vi "AddClassCase.vi"(2 "error in":errorcluster, 3 "Class path":path, 4 "CaseSel Refnum":refnum<vi>) -> (0 "error out":errorcluster, 1 "dup CaseSel Refnum":refnum<vi>)   [LabVIEW 2009, in "HGF_VisitorGenerator.lvlib"]
doc: "add case with default object of given class to factory's classes.vi"
uses:
  HGF_VisitorGenerator.lvlib
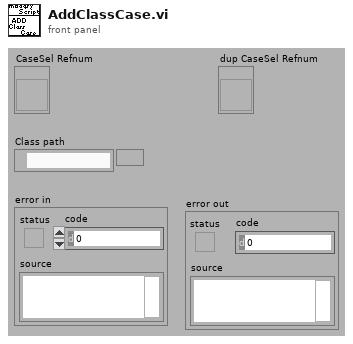
[diagram p1: front panel]
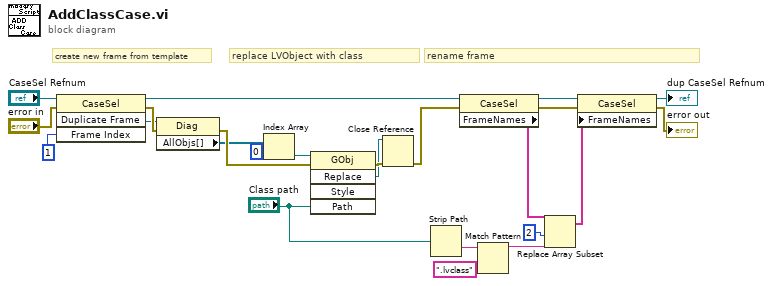
[diagram p0: block diagram]
diagram:
  # "rename frame"
  # "replace LVObject with class"
  # "create new frame from template"
  n1 = invoke class="CaseSel" method="Duplicate Frame"(reference="CaseSel Refnum", error in="error in", "Frame Index"=u32 1) -> (reference out=w8:refnum<vi>, error out=w23:errorcluster, "Duplicate Frame"=w21:refnum<vi>)  [unwired: 1 in, 1 out]
  n2 = property class="Diag"(reference=w21, error in=w23) -> (error out=w24:errorcluster, "AllObjs[]"=w15:refnum<vi>[])  [unwired: 1 out]
  n3 = Index Array(array=w15, index=0) -> (element=w14:refnum<vi>)
  n4 = invoke class="GObj" method="Replace"(reference=w14, error in=w24, "Path"="Class path") -> (error out=w18:errorcluster, "Replace"=w17:refnum<vi>)  [unwired: 2 in, 3 out]
  n5 = Close Reference(reference=w17, error in (no error)=w18) -> (error out=w6:errorcluster)
  n6 = Strip Path(path="Class path") -> (name=w12:string)  [unwired: 1 out]
  n7 = property class="CaseSel"(reference=w8, error in=w6) -> (reference out=w9:refnum<vi>, error out=w5:errorcluster, "FrameNames"=w3:string[])
  n8 = Match Pattern(string=w12, regular expression=".lvclass") -> (before substring=w13:string)  [unwired: 1 in, 3 out]
  n9 = Replace Array Subset(array=w3, new element=w13, index=2) -> (w10:string[])
  n10 = property class="CaseSel"(reference=w9, error in=w5, "FrameNames"=w10) -> (reference out=→"dup CaseSel Refnum":refnum<vi>, error out=→"error out":errorcluster)
